vi "ArmControlManual.vi"(7 "Extension Triggers":cluster{"Retract":dbl, "Extend":dbl}, 8 "error in (no error)":errorcluster, 9 "Pivot Stick":cluster{"X":dbl, "Y":dbl}, 10 "Wrist Stick":cluster{"Y":dbl, "X":dbl}) -> (0 "error out":errorcluster)   [LabVIEW 2014]
panel:
  in  "Wrist Multiplier":dbl=0.25 format="%#_13g"
  in  "Pivot Multiplier":dbl=0.25
  in  "Extension Multiplier":dbl=0.25
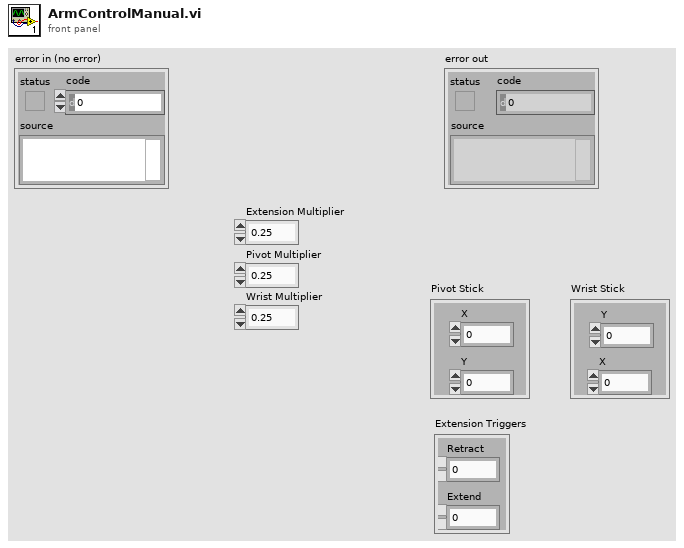
[diagram p1: front panel]
types:
  T1 = typedef "WPI_MotorControlDeviceRef.ctl" = cluster{"DeviceStatus":errorcluster, "Type":T2, "PWM":cluster{"Controller":T3, "PWM Channel":T4, "DeadBand":T5}, "CAN":cluster{"Device Number":u8, "Control Mode":T6, "Semaphore":T7, "Max Vout":dbl, "TalonSRX Control Mode":T8}, "Invert":bool, "TransformRef":T9, "InvTransformRef":T9}
  T2 = typedef "WPI_MotorControlType.ctl" = enum16{"PWM", "CAN", "CANTalonSRX"}
  T3 = typedef "FPGA_TypedefDigitalModule.ctl" = enum16{"Controller 1"}
  T4 = typedef "FPGA_DIOPWMChannel.ctl" = enum8{"PWM 0", "PWM 1", "PWM 2", "PWM 3", "PWM 4", "PWM 5", "PWM 6", "PWM 7", "PWM 8", "PWM 9", "PWM MXP 0", "PWM MXP 1", "PWM MXP 2", "PWM MXP 3", "PWM MXP 4", "PWM MXP 5", "PWM MXP 6", "PWM MXP 7", "PWM MXP 8", "PWM MXP 9", "Invalid"}
  T5 = typedef "WPI_PWMDeadband.ctl" = cluster{"Name":string, "maxPositivePwm":i32, "minPositivePwm":i32, "centerPwm":i32, "maxNegativePwm":i32, "minNegativePwm":i32, "angularRange":u16}
  T6 = typedef "WPI_CANJaguar_ControlMode.ctl" = enum8{"Percent VBus", "Current", "Speed", "Position", "Voltage"}
  T7 = typedef "Semaphore RefNum" = refnum<k1>
  T8 = typedef "WPI_CANTalonSRX_APIControlMode.ctl" = enum8{"Percent VBus", "Speed", "Position", "Slave", "Unchanged / Invalid"}
  T9 = typedef "WPI_PWMTransform_ConPane.ctl" = refnum<vi>
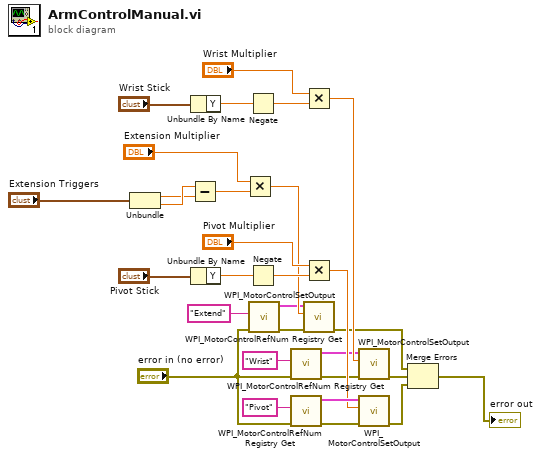
[diagram p0: block diagram]
diagram:
  n1 = Unbundle("Extension Triggers") -> ("Retract"=w9:dbl, "Extend"=w10:dbl)
  n2 = Subtract(x=w10, y=w9) -> (x-y=w8:dbl)
  n3 = Unbundle By Name("Wrist Stick") -> ("Y"=w16:dbl)
  n4 = Unbundle By Name("Pivot Stick") -> ("Y"=w25:dbl)
  n5 = Multiply(x="Extension Multiplier", y=w8) -> (x*y=w12:dbl)
  n6 = Negate(x=w16) -> (-x=w19:dbl)
  n7 = Negate(x=w25) -> (-x=w24:dbl)
  n8 = call <vilib>:"WPI_MotorControlRefNum Registry Get.vi"("error in (no error)"="error in (no error)", "refnum name"="Extend") -> ("error out"=w6:errorcluster, "MotorControlDevRef"=w5:T1)  [unwired: 8 in]
  n9 = call <vilib>:"WPI_MotorControlRefNum Registry Get.vi"("error in (no error)"="error in (no error)", "refnum name"="Wrist") -> ("error out"=w14:errorcluster, "MotorControlDevRef"=w13:T1)  [unwired: 8 in]
  n10 = call <vilib>:"WPI_MotorControlRefNum Registry Get.vi"("error in (no error)"="error in (no error)", "refnum name"="Pivot") -> ("error out"=w22:errorcluster, "MotorControlDevRef"=w23:T1)  [unwired: 8 in]
  n11 = Multiply(x="Wrist Multiplier", y=w19) -> (x*y=w18:dbl)
  n12 = Multiply(x="Pivot Multiplier", y=w24) -> (x*y=w21:dbl)
  n13 = call <vilib>:"WPI_MotorControlSetOutput.vi"("error in (no error)"=w6, "Output"=w12, "MotorControlDevRef"=w5) -> ("error out"=w2:errorcluster)  [unwired: 6 in, 2 out]
  n14 = call <vilib>:"WPI_MotorControlSetOutput.vi"("error in (no error)"=w14, "Output"=w18, "MotorControlDevRef"=w13) -> ("error out"=w4:errorcluster)  [unwired: 6 in, 2 out]
  n15 = call <vilib>:"WPI_MotorControlSetOutput.vi"("error in (no error)"=w22, "Output"=w21, "MotorControlDevRef"=w23) -> ("error out"=w1:errorcluster)  [unwired: 6 in, 2 out]
  n16 = Merge Errors(w2, w4, w1) -> (→"error out":errorcluster)
